vi "PDLM_GetLHData.vi"(8 "error in (no error)":errorcluster, 11 "USBIdx":i32) -> (0 "error out":errorcluster, 2 "Data":T1 {"LaserType" items=["UNDEFINED"=0, "LDH"=16, "LDH_FSL"=24, "LED"=32, "TA_SHG"=48, "FIBER"=64, "FIBER_FSL"=72, "FA"=80, "FA_SHG"=96, "BRIDGE"=240]}, 3 "return type":i32)   [LabVIEW 2019]
uses:
  <userlib>/TaikoLaser/PDLM_LHData.ctl
  <userlib>/TaikoLaser/PDLM_LHData_LaserType.ctl
  <userlib>/TaikoLaser/PDLM_LHVersion.ctl
  <userlib>/TaikoLaser/PDLM_DllPath_global.vi
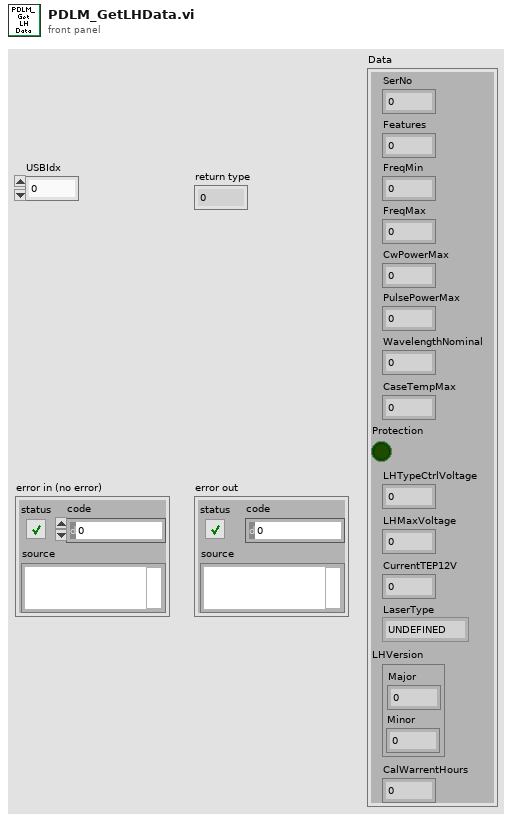
[diagram p1: front panel]
types:
  T1 = typedef "PDLM_LHData.ctl" = cluster{"SerNo":u32, "Features":u32, "FreqMin":u32, "FreqMax":u32, "CwPowerMax":u32, "PulsePowerMax":u32, "WavelengthNominal":u16, "CaseTempMax":u16, "Protection":bool, "LHTypeCtrlVoltage":u16, "LHMaxVoltage":u16, "CurrentTEP12V":u16, "LaserType":T2, "LHVersion":T3, "CalWarrentHours":u16}
  T2 = typedef "PDLM_LHData_LaserType.ctl" = u16
  T3 = typedef "PDLM_LHVersion.ctl" = cluster{"Major":u16, "Minor":u16}
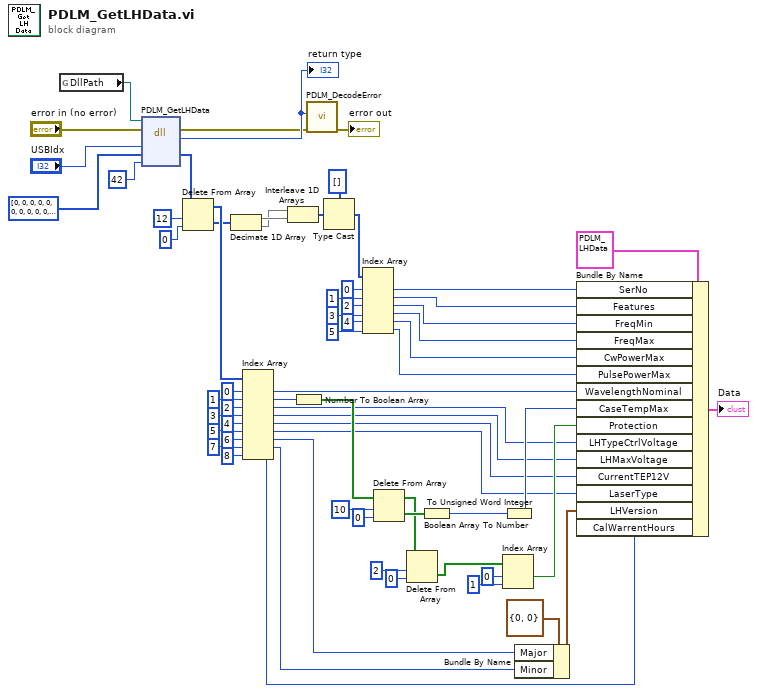
[diagram p0: block diagram]
diagram:
  n1 = global read "PDLM_DllPath_global.vi" "DllPath"() -> (w61:path)
  n2 = dll-call lib="M:/_dev/progs/LabVIEW/_lib/PQ/Taiko/pdlm_lib.dll" fn="PDLM_GetLHData"(path in=w61, error in="error in (no error)", "USBIdx"="USBIdx", "Data"=u16[] [0, 0, 0, 0, 0, 0, 0, 0, 0, 0, 0, 0, 0, 0, 0, 0, 0, 0, 0, 0, 0], "size"=u32 42) -> (error out=w63:errorcluster, "return type"=w64:i32, "Data"=w58:u16[])  [unwired: 3 in, 1 out]
  "return type" <- w64
  n3 = Delete From Array(array=w58, length=12, index=0) -> (deleted portion=w1:u16[], array with subset deleted=w40:u16[])
  n4 = Decimate 1D Array(w1) -> (w5:u16[], w4:u16[])
  n5 = Index Array(array=w40, index #1=0 ("index"), index #2=1 ("index"), index #3=2 ("index"), index #4=3 ("index"), index #5=4 ("index"), index #6=5 ("index"), index #7=6 ("index"), index #8=7 ("index"), index #9=8 ("index")) -> (element #1=w39:u16, element #2=w38:u16, element #3=w21:u16, element #4=w19:u16, element #5=w17:u16, element #6=w15:u16, element #7=w12:u16, element #8=w9:u16, element #9=w7:u16)
  n6 = Interleave 1D Arrays(w4, w5) -> (w3:u16[])
  n7 = Number To Boolean Array(number=w38) -> (Boolean array=w37:bool[])
  n8 = call <userlib>:"PDLM_DecodeError.vi"("error in (no error)"=w63, "code"=w64) -> ("error out"=→"error out":errorcluster)  [unwired: 7 in, 2 out]
  n9 = Type Cast(type=u32[] [], x=w3) -> (*(type *) &x=w2:u32[])
  n10 = Index Array(array=w2, index #1=0 ("index"), index #2=1 ("index"), index #3=2 ("index"), index #4=3 ("index"), index #5=4 ("index"), index #6=5 ("index")) -> (element #1=w52:u32, element #2=w51:u32, element #3=w50:u32, element #4=w49:u32, element #5=w48:u32, element #6=w47:u32)
  n11 = Delete From Array(array=w37, length=10, index=0) -> (deleted portion=w34:bool[], array with subset deleted=w27:bool[])
  n12 = Delete From Array(array=w27, length=2, index=0) -> (deleted portion=w26:bool[])  [unwired: 1 out]
  n13 = Boolean Array To Number(Boolean array=w34) -> (number=w33:u32)
  n14 = Index Array(array=w26, index #1=0 ("index"), index #2=1 ("index")) -> (element #1=w23:bool)  [unwired: 1 out]
  n15 = To Unsigned Word Integer(number=w33) -> (unsigned 16bit integer=w32:u16)
  n16 = Bundle By Name(cluster=T3 {"Major"=0, "Minor"=0} ("PDLM_LHVersion"), "Major"=w12, "Minor"=w9) -> (w8:T3)
  n17 = Bundle By Name(cluster=T1 {"SerNo"=0, "Features"=0, "FreqMin"=0, "FreqMax"=0, "CwPowerMax"=0, "PulsePowerMax"=0, "WavelengthNominal"=0, "CaseTempMax"=0, "Protection"=FALSE, "LHTypeCtrlVoltage"=0, "LHMaxVoltage"=0, "CurrentTEP12V"=0, "LaserType"=0, "LHVersion"={"Major"=0, "Minor"=0}, "CalWarrentHours"=0} ("LHData"), "SerNo"=w52, "Features"=w51, "FreqMin"=w50, "FreqMax"=w49, "CwPowerMax"=w48, "PulsePowerMax"=w47, "WavelengthNominal"=w39, "CaseTempMax"=w32, "Protection"=w23, "LHTypeCtrlVoltage"=w21, "LHMaxVoltage"=w19, "CurrentTEP12V"=w17, "LaserType"=w15, "LHVersion"=w8, "CalWarrentHours"=w7) -> (→"Data":T1)
